vi "set BK9129B enable x3.vi"(0 "ch 1 state":bool, 1 "ch 2 state":bool, 2 "ch 3 state":bool, 3 "error in":errorcluster, 4 "VISA in":refnum<visa-resource-name>="GPIB0::12::INSTR") -> (5 "VISA out":refnum<visa-resource-name>="GPIB0::12::INSTR", 6 "error out":errorcluster)   [LabVIEW 2018]
panel:
  out "output string":string
  # "inputs"
  # "outputs"
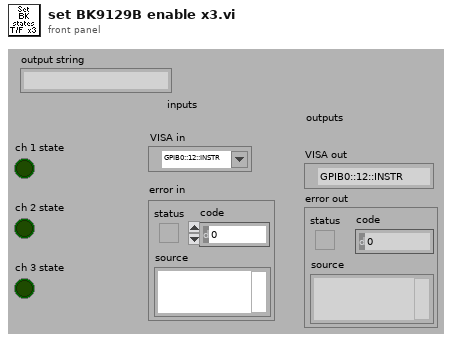
[diagram p1: front panel]
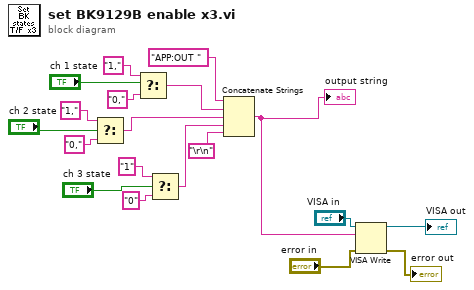
[diagram p0: block diagram]
diagram:
  n1 = Select(t="1," ("format string"), s="ch 2 state", f="0," ("format string")) -> (s? t:f=w2:string)
  n2 = Select(t="1," ("format string"), s="ch 1 state", f="0," ("format string")) -> (s? t:f=w3:string)
  n3 = Select(t="1" ("format string"), s="ch 3 state", f="0" ("format string")) -> (s? t:f=w1:string)
  n4 = Concatenate Strings("APP:OUT " ("format string"), w3, w2, w1, "\r\n") -> (w17:string)
  "output string" <- w17
  n5 = VISA Write(VISA resource name="VISA in", write buffer=w17, error in (no error)="error in") -> (VISA resource name out=→"VISA out":refnum<visa-resource-name>, error out=→"error out":errorcluster)  [unwired: 1 out]
